vi "Atto DRY Interface get Attodry Error Status.vi"(8 "error in (no error)":errorcluster, 11 "ErrorCode":string) -> (0 "error out":errorcluster, 2 "function return":i32, 3 "ErrorCode out":string)   [LabVIEW 2016, in "attoDRYLib.lvlib"]
doc: "int32_t __cdecl AttoDRY_Interface_getAttodryErrorStatus(uint8_t *ErrorCode);"
uses:
  <userlib>/attoDRYLib/attoDRYLib.lvlib
  <userlib>/attoDRYLib/attoDRYLib.dll
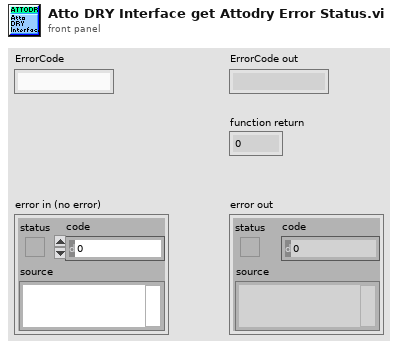
[diagram p1: front panel]
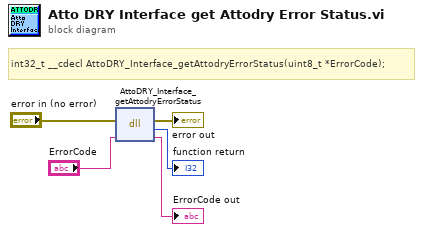
[diagram p0: block diagram]
diagram:
  # "int32_t __cdecl AttoDRY_Interface_getAttodryErrorStatus(uint8_t *ErrorCode);"
  n1 = dll-call lib="C:/Program Files (x86)/National Instruments/LabVIEW 2016/user.lib/attoDRYLib/attoDRYLib.*" fn="AttoDRY_Interface_getAttodryErrorStatus"(error in="error in (no error)", "ErrorCode"="ErrorCode") -> (error out=→"error out":errorcluster, →"function return":i32, "ErrorCode"=→"ErrorCode out":string)  [unwired: 2 in, 1 out]
